vi "Z Aux Get Modbus Dpos.vi"(8 "error in (no error)":errorcluster caption="错误输入（无错误）", 9 "pValueList":sgl[](array[numeric])=array[4097 elements], 10 "imaxaxises":i32, 11 "handle":u32) -> (0 "error out":errorcluster caption="错误输出", 1 "pValueList out":sgl[](array[numeric]), 2 "function return":i32, 3 "handle out":u32)   [LabVIEW 2015, in "zauxdll.lvlib"]
doc: "int32 __stdcall ZAux_GetModbusDpos(ZMC_HANDLE handle, int imaxaxises, float pValueList[]);"
uses:
  zauxdll.lvlib
  Radar - 2015 32bit_autoqueue_angle_0319/zauxdll-2014/zauxdll.dll
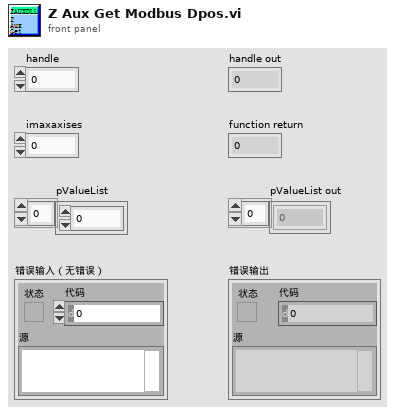
[diagram p1: front panel]
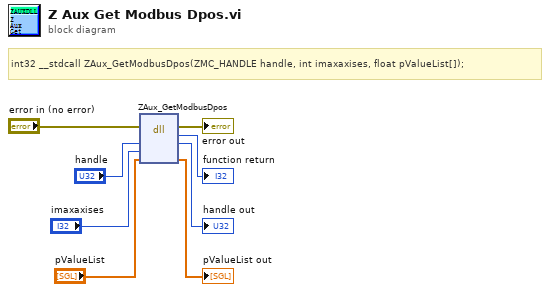
[diagram p0: block diagram]
diagram:
  # "int32 __stdcall ZAux_GetModbusDpos(ZMC_HANDLE handle, int imaxaxises, float pValueList[]);"
  n1 = dll-call lib="D:/vicomm case/cub/0717/Radar - 2015 32bit_autoqueue_angle_0319/zauxdll-2014/zauxdll.*" fn="ZAux_GetModbusDpos"(error in="error in (no error)", "handle"="handle", "imaxaxises"="imaxaxises", "pValueList"="pValueList") -> (error out=→"error out":errorcluster, →"function return":i32, "handle"=→"handle out":u32, "pValueList"=→"pValueList out":sgl[])  [unwired: 3 in, 1 out]
